vi "1 UpdateChartData.vi"(8 "error in (no error)":errorcluster caption="错误输入（无错误）", 11 "Chart Actor 输入":refnum<class "Chart Actor.lvclass">) -> (0 "error out":errorcluster caption="错误输出", 3 "Chart Actor 输出":refnum<class "Chart Actor.lvclass">)   [LabVIEW 2018, in "Chart Actor.lvlib" / "Chart Actor.lvclass"]
uses:
  Chart Actor.lvclass
  Chart Actor.lvclass/Chart Actor.ctl
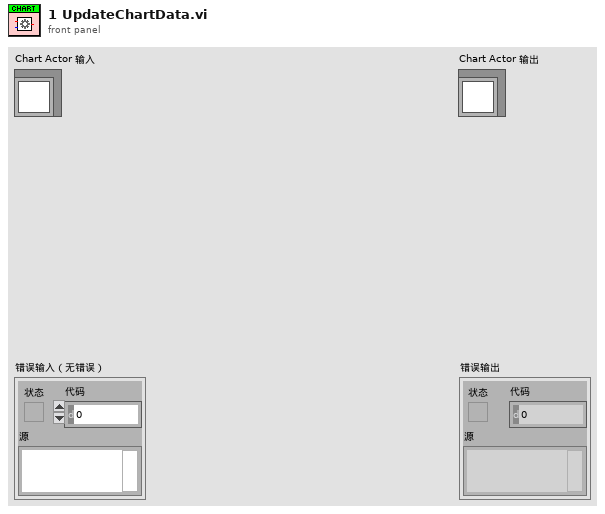
[diagram p1: front panel]
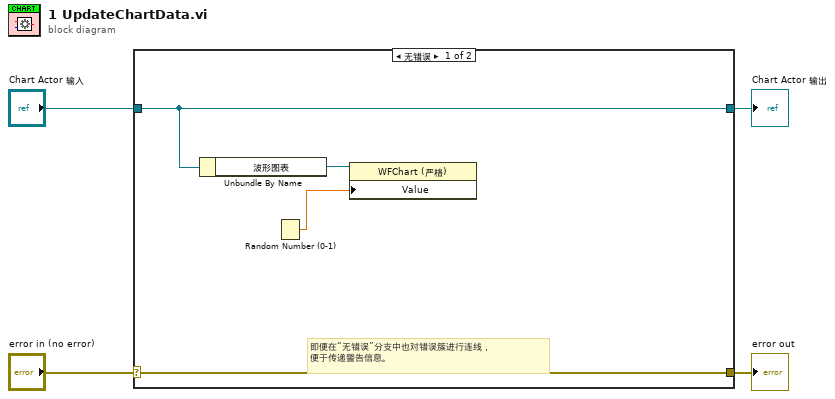
[diagram p0: block diagram]
diagram:
  n1 = case shown="无错误" "error in (no error)" {
    selector: "error in (no error)" -> [w8 w10]
    tunnel: [w8 w10] -> w3
    tunnel: [w7 w9] -> w1
    tunnel: "Chart Actor 输入" -> [w7 w9]
    frame No Error {
      # "即便在“无错误”分支中也对错误簇进行连线，\n便于传递警告信息。"
      n2 = Unbundle By Name(w7) -> ("波形图表"=w6:refnum<vi>)
      n3 = Random Number (0-1)() -> (number: 0 to 1=w5:dbl)
      n4 = property class="WFChart (严格)"(reference=w6, "Value"=w5) -> ()  [unwired: 1 in, 2 out]
    }
    frame Error {
    }
  }
  "error out" <- w3
  "Chart Actor 输出" <- w1
